vi "Optical Pulse Sequence Generator with sig pulse only.vi"(6 "N Loop":i32=25000, 8 "AOM Rest time":dbl, 9 "Signal delay":dbl, 10 "APD signal width":dbl, 11 "AOM Pulse length":dbl=3e-07) -> (0 "Array":T1(array[cluster]), 3 "No. Instructions":i32)   [LabVIEW 2012]
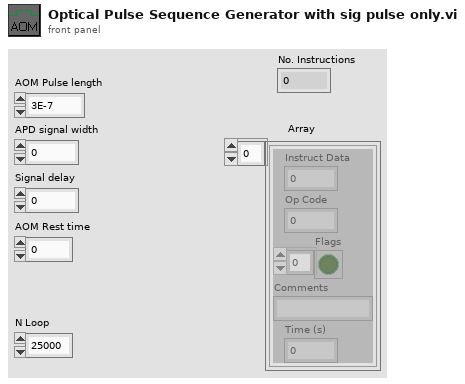
[diagram p1: front panel]
types:
  T1 = cluster{"Instruct Data":i32, "Op Code":i32, "Flags":bool[], "Comments":string, "Time (s)":dbl}[]
  T2 = cluster{"Instruct Data":i32, "Op Code":i32, "Flags":bool[], "Comments":string, "Time (s)":dbl}
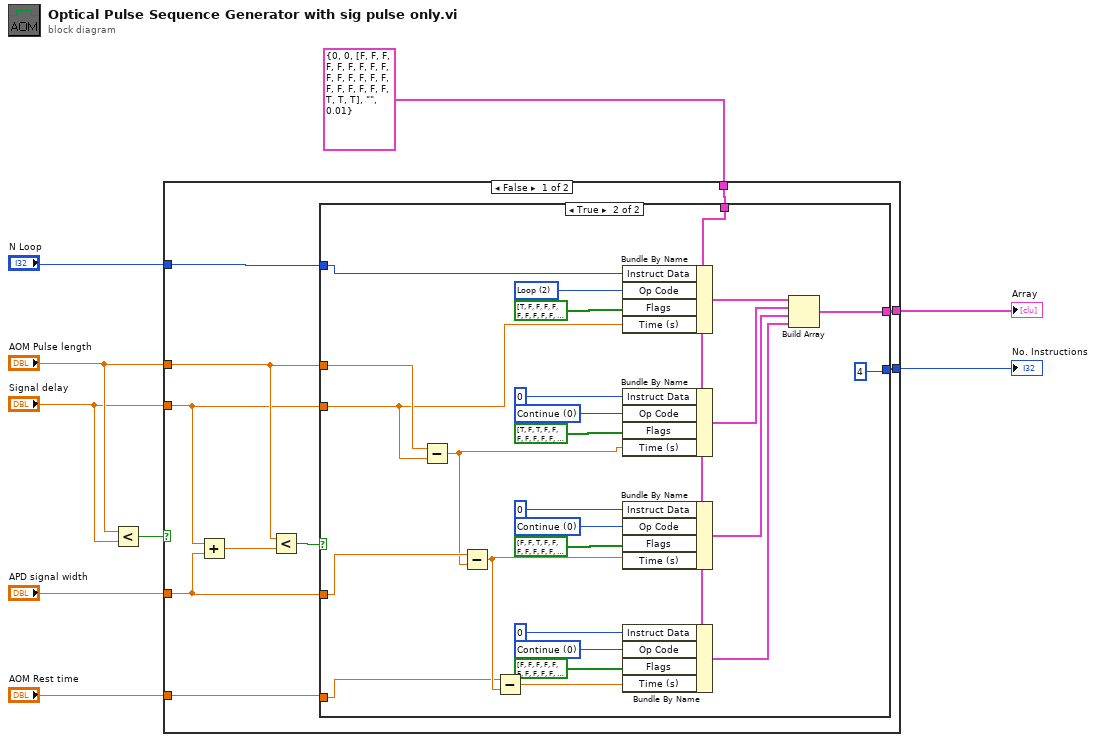
[diagram p0: block diagram]
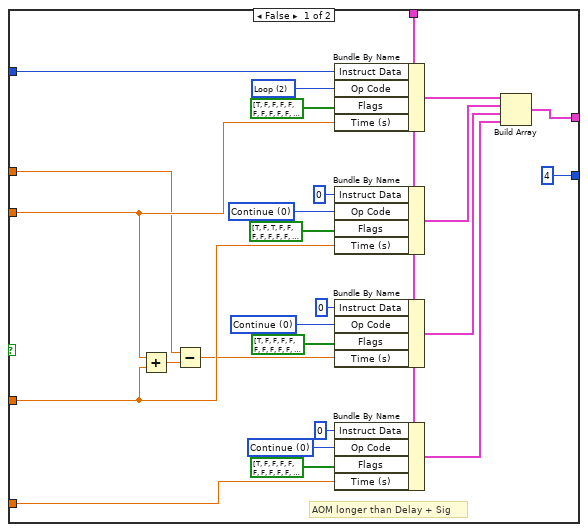
[diagram p2: hidden frame]
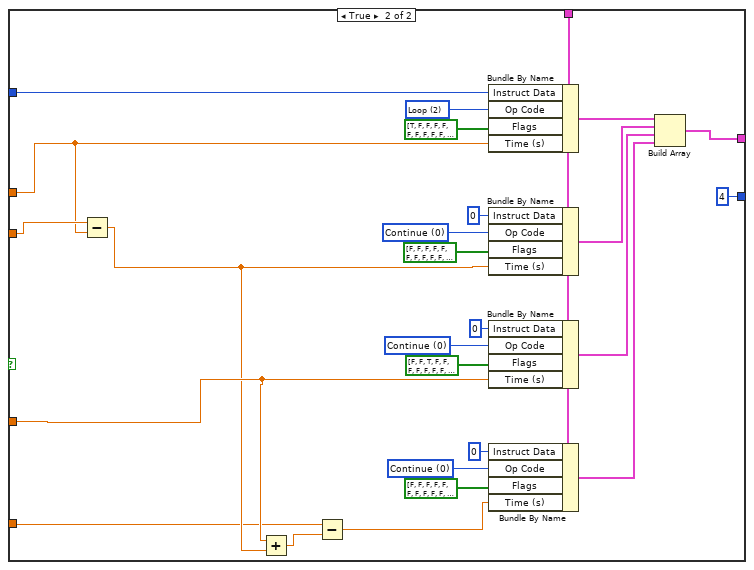
[diagram p3: hidden frame]
diagram:
  n1 = Less?(x="AOM Pulse length", y="Signal delay") -> (x < y?=w9:bool)
  n2 = case shown="False" w9 {
    tunnel: "AOM Pulse length" -> [w16 w76]
    tunnel: "Signal delay" -> [w10 w77]
    tunnel: "APD signal width" -> [w12 w75]
    tunnel: "AOM Rest time" -> [w15 w72]
    tunnel: T2 {"Instruct Data"=0, "Op Code"=0, "Flags"=[FALSE, FALSE, FALSE, FALSE, FALSE, FALSE, FALSE, FALSE, FALSE, FALSE, FALSE, FALSE, FALSE, FALSE, FALSE, FALSE, FALSE, FALSE, FALSE, FALSE, FALSE, TRUE, TRUE, TRUE], "Comments"="", "Time (s)"=0.01} ("PB Inst 2") -> [w18 w80]
    tunnel: "N Loop" -> [w17 w81]
    tunnel: [w14 w79] -> w2
    tunnel: [w13 4] -> w1
    frame False {
      n3 = Add(x=w10, y=w12) -> (x+y=w11:dbl)
      n4 = Less?(x=w16, y=w11) -> (x < y?=w19:bool)
      n5 = case shown="True" w19 {
        tunnel: w18 -> [w32 w55]
        tunnel: w17 -> [w42 w52]
        tunnel: w16 -> [w22 w51]
        tunnel: w10 -> [w24 w50]
        tunnel: w12 -> [w25 w49]
        tunnel: w15 -> [w20 w46]
        tunnel: [w27 w53] -> w14
        tunnel: [4 4] -> w13
        frame False {
          w34 = 0 items=["Continue", "Stop", "Loop", "End Loop", "JSR", "RTS", "Branch", "Long Delay", "Wait"] ("Op Code")
          w37 = 0 items=["Continue", "Stop", "Loop", "End Loop", "JSR", "RTS", "Branch", "Long Delay", "Wait"] ("Op Code")
          w40 = 0 items=["Continue", "Stop", "Loop", "End Loop", "JSR", "RTS", "Branch", "Long Delay", "Wait"] ("Op Code")
          w43 = 2 items=["Continue", "Stop", "Loop", "End Loop", "JSR", "RTS", "Branch", "Long Delay", "Wait"] ("Op Code")
          # "AOM longer than Delay + Sig"
          n6 = Add(x=w24, y=w25) -> (x+y=w23:dbl)
          n7 = Subtract(x=w22, y=w23) -> (x-y=w21:dbl)
          n8 = Bundle By Name(cluster=w32, "Instruct Data"=w42, "Op Code"=w43, "Flags"=bool[] [TRUE, FALSE, FALSE, FALSE, FALSE, FALSE, FALSE, FALSE, FALSE, FALSE, FALSE, FALSE, FALSE, FALSE, FALSE, FALSE, FALSE, FALSE, FALSE, FALSE, FALSE, TRUE, TRUE, TRUE], "Time (s)"=w24) -> (w31:T2)
          n9 = Bundle By Name(cluster=w32, "Instruct Data"=0, "Op Code"=w40, "Flags"=bool[] [TRUE, FALSE, TRUE, FALSE, FALSE, FALSE, FALSE, FALSE, FALSE, FALSE, FALSE, FALSE, FALSE, FALSE, FALSE, FALSE, FALSE, FALSE, FALSE, FALSE, FALSE, TRUE, TRUE, TRUE], "Time (s)"=w25) -> (w28:T2)
          n10 = Bundle By Name(cluster=w32, "Instruct Data"=0, "Op Code"=w37, "Flags"=bool[] [TRUE, FALSE, FALSE, FALSE, FALSE, FALSE, FALSE, FALSE, FALSE, FALSE, FALSE, FALSE, FALSE, FALSE, FALSE, FALSE, FALSE, FALSE, FALSE, FALSE, FALSE, TRUE, TRUE, TRUE], "Time (s)"=w21) -> (w29:T2)
          n11 = Bundle By Name(cluster=w32, "Instruct Data"=0, "Op Code"=w34, "Flags"=bool[] [TRUE, FALSE, FALSE, FALSE, FALSE, FALSE, FALSE, FALSE, FALSE, FALSE, FALSE, FALSE, FALSE, FALSE, FALSE, FALSE, FALSE, FALSE, FALSE, FALSE, FALSE, TRUE, TRUE, TRUE], "Time (s)"=w20) -> (w30:T2)
          n12 = Build Array(w31, w28, w29, w30) -> (w27:T1)
        }
        frame True {
          w61 = 0 items=["Continue", "Stop", "Loop", "End Loop", "JSR", "RTS", "Branch", "Long Delay", "Wait"] ("Op Code")
          w64 = 0 items=["Continue", "Stop", "Loop", "End Loop", "JSR", "RTS", "Branch", "Long Delay", "Wait"] ("Op Code")
          w67 = 0 items=["Continue", "Stop", "Loop", "End Loop", "JSR", "RTS", "Branch", "Long Delay", "Wait"] ("Op Code")
          w69 = 2 items=["Continue", "Stop", "Loop", "End Loop", "JSR", "RTS", "Branch", "Long Delay", "Wait"] ("Op Code")
          n13 = Subtract(x=w51, y=w50) -> (x-y=w48:dbl)
          n14 = Subtract(x=w49, y=w48) -> (x-y=w47:dbl)
          n15 = Subtract(x=w46, y=w47) -> (x-y=w45:dbl)
          n16 = Bundle By Name(cluster=w55, "Instruct Data"=w52, "Op Code"=w69, "Flags"=bool[] [TRUE, FALSE, FALSE, FALSE, FALSE, FALSE, FALSE, FALSE, FALSE, FALSE, FALSE, FALSE, FALSE, FALSE, FALSE, FALSE, FALSE, FALSE, FALSE, FALSE, FALSE, TRUE, TRUE, TRUE], "Time (s)"=w50) -> (w59:T2)
          n17 = Bundle By Name(cluster=w55, "Instruct Data"=0, "Op Code"=w67, "Flags"=bool[] [TRUE, FALSE, TRUE, FALSE, FALSE, FALSE, FALSE, FALSE, FALSE, FALSE, FALSE, FALSE, FALSE, FALSE, FALSE, FALSE, FALSE, FALSE, FALSE, FALSE, FALSE, TRUE, TRUE, TRUE], "Time (s)"=w48) -> (w56:T2)
          n18 = Bundle By Name(cluster=w55, "Instruct Data"=0, "Op Code"=w64, "Flags"=bool[] [FALSE, FALSE, TRUE, FALSE, FALSE, FALSE, FALSE, FALSE, FALSE, FALSE, FALSE, FALSE, FALSE, FALSE, FALSE, FALSE, FALSE, FALSE, FALSE, FALSE, FALSE, TRUE, TRUE, TRUE], "Time (s)"=w47) -> (w57:T2)
          n19 = Bundle By Name(cluster=w55, "Instruct Data"=0, "Op Code"=w61, "Flags"=bool[] [FALSE, FALSE, FALSE, FALSE, FALSE, FALSE, FALSE, FALSE, FALSE, FALSE, FALSE, FALSE, FALSE, FALSE, FALSE, FALSE, FALSE, FALSE, FALSE, FALSE, FALSE, TRUE, TRUE, TRUE], "Time (s)"=w45) -> (w58:T2)
          n20 = Build Array(w59, w56, w57, w58) -> (w53:T1)
        }
      }
    }
    frame True {
      w91 = 0 items=["Continue", "Stop", "Loop", "End Loop", "JSR", "RTS", "Branch", "Long Delay", "Wait"] ("Op Code")
      w88 = 0 items=["Continue", "Stop", "Loop", "End Loop", "JSR", "RTS", "Branch", "Long Delay", "Wait"] ("Op Code")
      w85 = 0 items=["Continue", "Stop", "Loop", "End Loop", "JSR", "RTS", "Branch", "Long Delay", "Wait"] ("Op Code")
      w83 = 2 items=["Continue", "Stop", "Loop", "End Loop", "JSR", "RTS", "Branch", "Long Delay", "Wait"] ("Op Code")
      n21 = Subtract(x=w77, y=w76) -> (x-y=w74:dbl)
      n22 = Add(x=w75, y=w74) -> (x+y=w73:dbl)
      n23 = Subtract(x=w72, y=w73) -> (x-y=w71:dbl)
      n24 = Bundle By Name(cluster=w80, "Instruct Data"=w81, "Op Code"=w83, "Flags"=bool[] [TRUE, FALSE, FALSE, FALSE, FALSE, FALSE, FALSE, FALSE, FALSE, FALSE, FALSE, FALSE, FALSE, FALSE, FALSE, FALSE, FALSE, FALSE, FALSE, FALSE, FALSE, TRUE, TRUE, TRUE], "Time (s)"=w76) -> (w93:T2)
      n25 = Bundle By Name(cluster=w80, "Instruct Data"=0, "Op Code"=w85, "Flags"=bool[] [FALSE, FALSE, FALSE, FALSE, FALSE, FALSE, FALSE, FALSE, FALSE, FALSE, FALSE, FALSE, FALSE, FALSE, FALSE, FALSE, FALSE, FALSE, FALSE, FALSE, FALSE, TRUE, TRUE, TRUE], "Time (s)"=w74) -> (w96:T2)
      n26 = Bundle By Name(cluster=w80, "Instruct Data"=0, "Op Code"=w88, "Flags"=bool[] [FALSE, FALSE, TRUE, FALSE, FALSE, FALSE, FALSE, FALSE, FALSE, FALSE, FALSE, FALSE, FALSE, FALSE, FALSE, FALSE, FALSE, FALSE, FALSE, FALSE, FALSE, TRUE, TRUE, TRUE], "Time (s)"=w75) -> (w95:T2)
      n27 = Bundle By Name(cluster=w80, "Instruct Data"=0, "Op Code"=w91, "Flags"=bool[] [FALSE, FALSE, FALSE, FALSE, FALSE, FALSE, FALSE, FALSE, FALSE, FALSE, FALSE, FALSE, FALSE, FALSE, FALSE, FALSE, FALSE, FALSE, FALSE, FALSE, FALSE, TRUE, TRUE, TRUE], "Time (s)"=w71) -> (w94:T2)
      n28 = Build Array(w93, w96, w95, w94) -> (w79:T1)
    }
  }
  "Array" <- w2
  "No. Instructions" <- w1
